vi "_Main.vi"() -> ()   [LabVIEW 2021]
uses:
  DemoApplication/DemoApplication.lvclass
  C:/Localdata/Projects/TriekselSoft/TriekselsoftApplicationFramework/Source/.Externals/Library_TAF_ApplicationFramework/MasterGUI/MasterGUI.lvclass
  .Externals/Library_TAF_ApplicationFramework/AppConfigJSON/AppConfigJSON.lvclass
  C:/Localdata/Projects/TriekselSoft/TriekselsoftApplicationFramework/Source/.Externals/Interface_TAF_IApplicationConfiguration/IApplicationConfiguration/IApplicationConfiguration.lvclass
  ErrorCreationTAF/ErrorCreationTAF.lvclass
  C:/Program Files (x86)/National Instruments/LabVIEW 2021/user.lib/_express/CustomErrorCreator/Source/ErrorCreationExecution/ErrorCreationExecution.lvclass
  .Externals/Library_TAF_TraceWindow/TraceWindow/TraceWindow.lvclass
  6e61f7a2-c992-4aa1-b06a-6e8223df94bd.vi
  cb46c3f9-39da-4d3f-bc1e-01bea614d4a3.vi
  deb2eb14-18af-4d58-82fc-a6efaabd3830.vi
  <vilib>/TriekselSoft/TracerLibrary/TracerLibrary/Tracer/protected/SendMessage.vi
  <vilib>/TriekselSoft/TracerLibrary/TracerLibrary/Tracer/protected/Timestamp.vi
  <vilib>/TriekselSoft/TracerLibrary/TracerLibrary/Tracer/Tracer_Level-Info.vi
  <vilib>/TriekselSoft/TracerLibrary/TracerLibrary/Tracer/protected/Tracer_ClassAttributes.vi
  <vilib>/TriekselSoft/TracerLibrary/TracerLibrary/Tracer/Tracer_Level-Error.vi
  .Externals/Library_TAF_ApplicationFramework/MasterGUI/MasterGUI.lvclass
  .Externals/Library_TAF_ApplicationFramework/Application/Application.lvclass
  <vilib>/TriekselSoft/TracerLibrary/TracerLibrary/Tracer/Tracer.lvclass
  <userlib>/_express/CustomErrorCreator/Source/ErrorCreationExecution/ErrorCreationExecution.lvclass
panel:
  in  "Configuration":enum16{"Default", "Mockup"}(ring)=enum."Mockup"
  out "Version":string
  out "Action":string
  out "Progress":dbl(slide) scale=0.0..1.0
  # "Application Template"
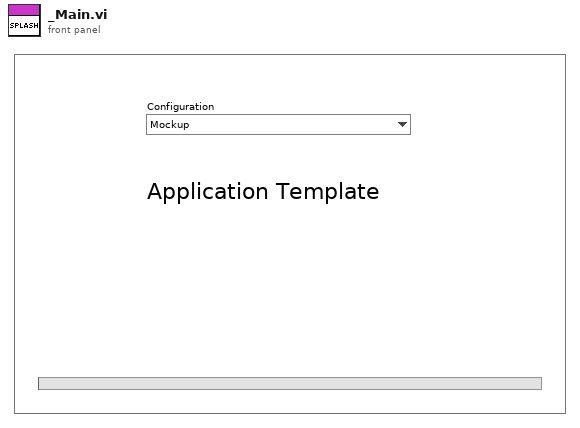
[diagram p1: front panel]
types:
  T1 = enum32{"Invalid", "Standard", "Closed", "Hidden", "Minimized", "Maximized"}
  T2 = enum32{"---START APPLICATION---", "Set Version", "Start Tracing", "Init Application", "Preload Objects", "Update Trace Items", "Create Objects", "Set External Interfaces", "Start Main GUI", "Load Presistent Data", "Show Main Window", "Hide Window", "Wait for Exit", "Save Persistent Data", "Show Window", "---EXIT APPLICATION---"}
  T3 = cluster{"DemoApplication":refnum<class "DemoApplication.lvclass">, "TraceQueue":refnum<queue>}
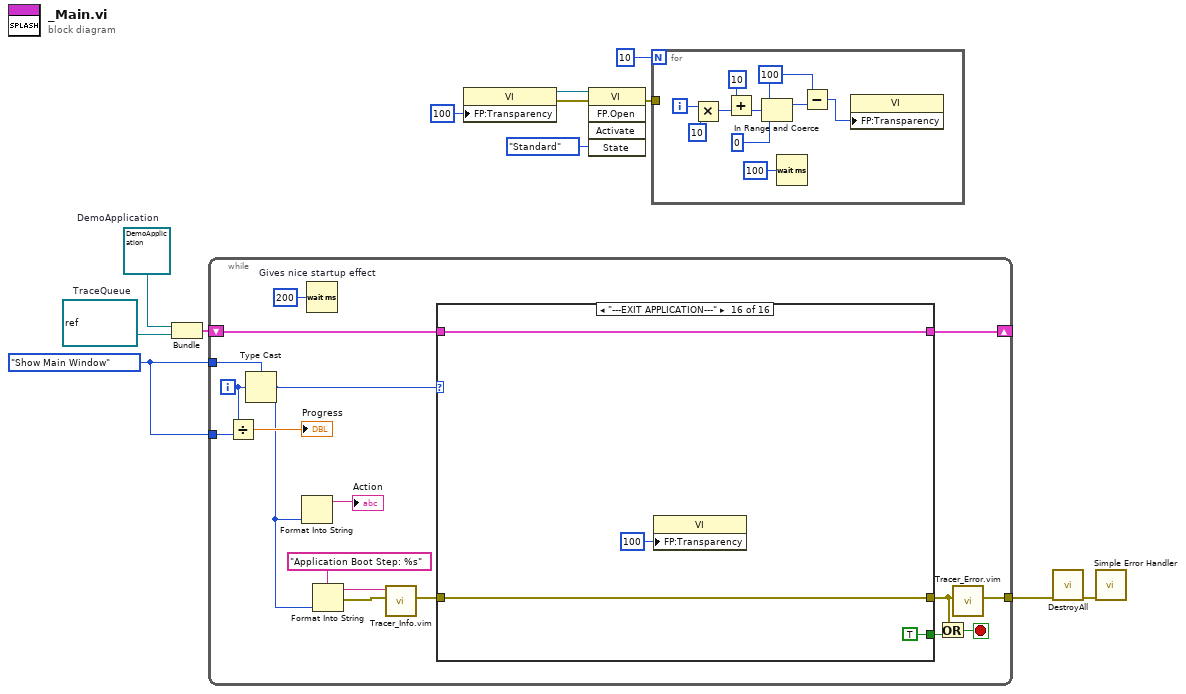
[diagram p0: block diagram]
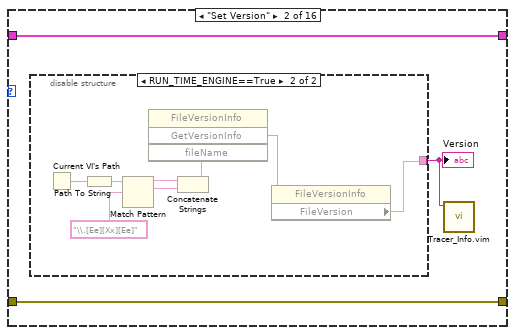
[diagram p3: hidden frame]
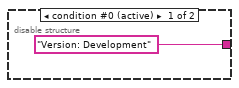
[diagram p4: hidden frame]
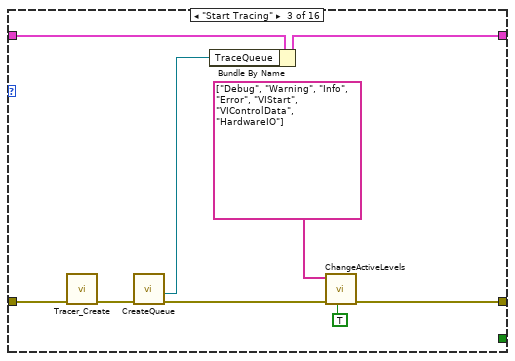
[diagram p5: hidden frame]
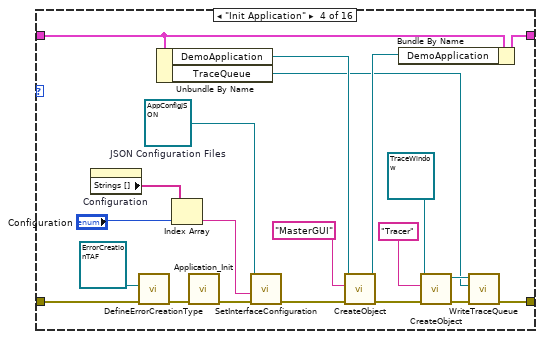
[diagram p6: hidden frame]
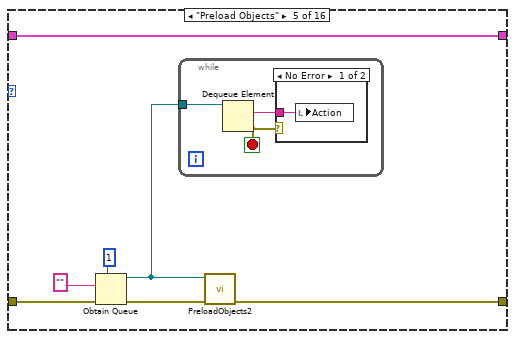
[diagram p7: hidden frame]
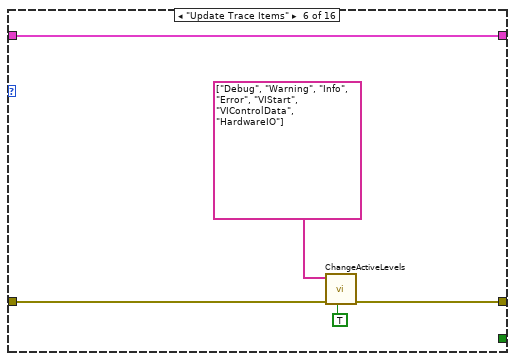
[diagram p9: hidden frame]
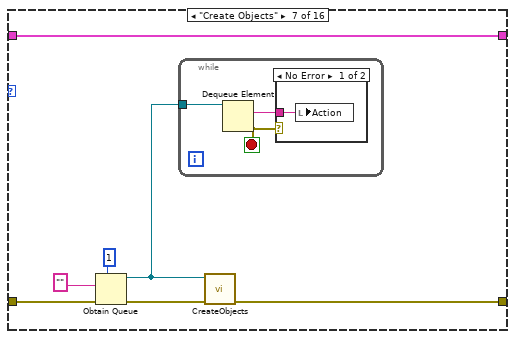
[diagram p10: hidden frame]
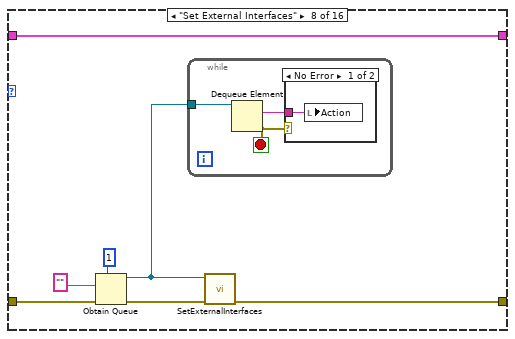
[diagram p12: hidden frame]
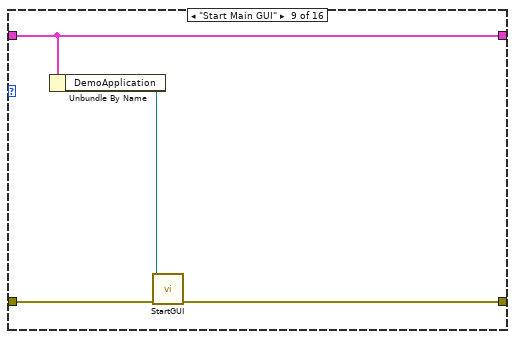
[diagram p14: hidden frame]
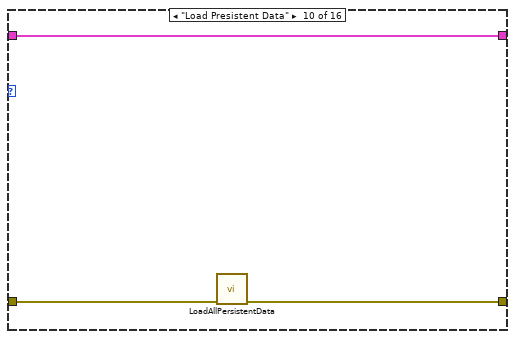
[diagram p15: hidden frame]
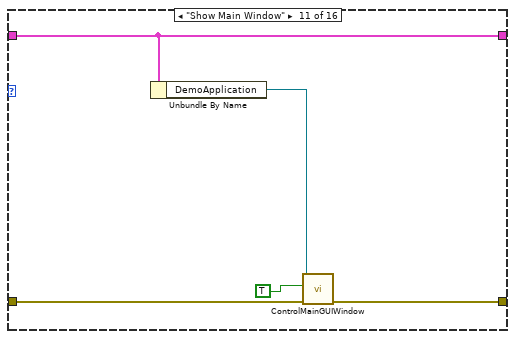
[diagram p16: hidden frame]
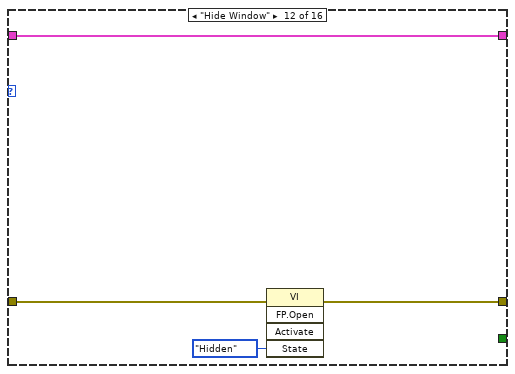
[diagram p17: hidden frame]
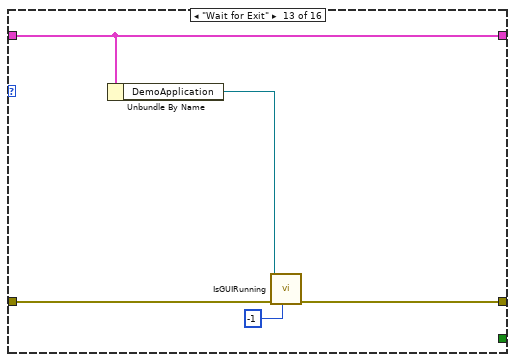
[diagram p18: hidden frame]
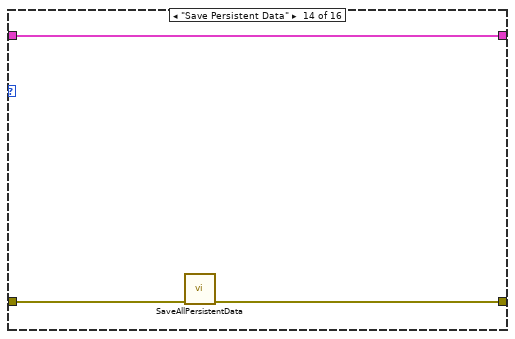
[diagram p19: hidden frame]
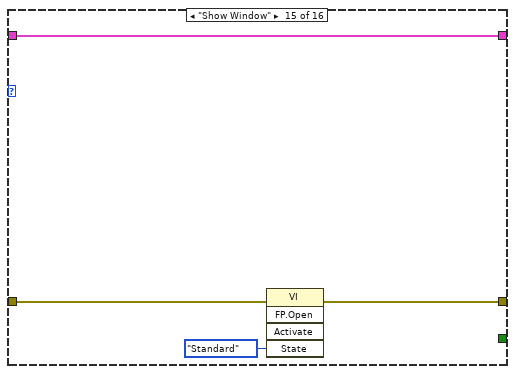
[diagram p20: hidden frame]
diagram:
  w1 = refnum<queue> refnum  # TraceQueue
  w3 = refnum<class "DemoApplication.lvclass"> refnum  # DemoApplication
  w4 = T2."Show Main Window"
  n1 = Bundle("DemoApplication"=w3, "TraceQueue"=w1) -> (w2:T3)  [unwired: 1 in]
  n2 = while {
    tunnel: w4 -> [w25]
    shift-right: [w21] -> _
    shift-left: w2 -> [w22]
    tunnel: [w28] -> w11
    tunnel: w4 -> [w15]
    i -> [w18]
    stop <- w20 stop-if-true
    n3 = Divide(x=w18, y=w15) -> (x/y=→"Progress":dbl)
    n4 = Type Cast(type=w25, x=w18) -> (*(type *) &x=w13:T2)
    n5 = Format Into String(w13) -> (resulting string=→"Action":string)  [unwired: 3 in, 1 out]
    n6 = Wait (ms) "Gives nice startup effect"(milliseconds to wait=u32 200) -> ()  [unwired: 1 out]
    n7 = Format Into String(format string="Application Boot Step: %s" ("InfoText"), w13) -> (resulting string=w23:string, error out=w27:errorcluster)  [unwired: 2 in]
    n8 = call "Tracer_Info.vim"("error in (no error)"=w27, "InfoText"=w23) -> ("error out"=w29:errorcluster)  [unwired: 9 in]
    n9 = case shown="\"---EXIT APPLICATION---\"" w13 {
      tunnel: w29 -> [w31 w34 w51 w71 w79 w88 w95 w106 w115 w118 w122 w127 w132 w135 w139 w143]
      tunnel: w22 -> [w30 w33 w46 w59 w77 w85 w93 w104 w112 w116 w120 w125 w129 w133 w137 w142]
      tunnel: [w30 w33 w45 w57 w77 w85 w93 w104 w112 w116 w120 w125 w129 w133 w137 w142] -> w21
      tunnel: [_ _ _ _ _ _ _ _ _ _ _ _ _ _ _ TRUE] -> w19
      tunnel: [w31 w34 w52 w67 w80 w89 w96 w107 w114 w117 w123 w126 w131 w134 w138 w143] -> w26
      frame "---START APPLICATION---" {
      }
      frame "Set Version" {
        n10 = disable-structure shown="RUN_TIME_ENGINE==True" {
          disable-tunnel: ["Version: Development" w36] -> w32
          frame condition #0 (active) {
          }
          frame condition #1 {
            n11 = Current VI's Path() -> (path=w39:path)
            n12 = Path To String(path=w39) -> (string=w43:string)
            n13 = Match Pattern(string=w43, regular expression="\\.[Ee][Xx][Ee]") -> (before substring=w41:string, match substring=w40:string)  [unwired: 1 in, 2 out]
            n14 = Concatenate Strings(w41, w40) -> (w42:string)
            n15 = invoke class="FileVersionInfo" method="GetVersionInfo"("fileName"=w42) -> ("GetVersionInfo"=w38:refnum<k24>)  [unwired: 3 in, 3 out]
            n16 = property class="FileVersionInfo"(reference=w38) -> ("FileVersion"=w36:string)  [unwired: 1 in, 2 out]
          }
        }
        "Version" <- w32
        n17 = call "Tracer_Info.vim"("InfoText"=w32) -> ()  [unwired: 10 in, 1 out]
      }
      frame "Start Tracing" {
        n18 = call <vilib>:"Tracer_Create.vi"("error in (no error)"=w51) -> ("error out"=w50:errorcluster)  [unwired: 10 in]
        n19 = call <vilib>:"CreateQueue.vi"("error in (no error)"=w50) -> ("error out"=w49:errorcluster, "Trace out"=w44:refnum<queue>)  [unwired: 9 in]
        n20 = Bundle By Name(cluster=w46, "TraceQueue"=w44) -> (w45:T3)
        n21 = call <vilib>:"ChangeActiveLevels.vi"("Force update"=TRUE, "error in (no error)"=w49, "ActiveLevels"=string[] ["Debug", "Warning", "Info", "Error", "VIStart", "VIControlData", "HardwareIO"] ("Active Compressed in")) -> ("error out"=w52:errorcluster)  [unwired: 8 in]
      }
      frame "Init Application" {
        w66 = refnum<class "AppConfigJSON.lvclass"> refnum  # JSON Configuration Files
        n22 = property on="Configuration" class="Enum (strict)"() -> ("Strings []"=w65:string[])  [unwired: 2 in, 2 out]
        n23 = call <userlib>:"DefineErrorCreationType.vi"("ErrorIn"=w71, "ErrorHandlingTypeClass"=refnum<class "ErrorCreationTAF.lvclass"> refnum ("ErrorCreationTAF")) -> ("ErrorOut"=w70:errorcluster)  [unwired: 9 in]
        n24 = Unbundle By Name(w59) -> ("DemoApplication"=w60:refnum<class "DemoApplication.lvclass">, "TraceQueue"=w53:refnum<queue>)
        n25 = Index Array(array=w65, index="Configuration") -> (element=w63:string)
        n26 = call "Application_Init.vi"("ErrorIn"=w70) -> ("ErrorOut"=w73:errorcluster)  [unwired: 9 in, 1 out]
        n27 = call "SetInterfaceConfiguration.vi"("ErrorIn"=w73, "StartupConfiguration"=w63, "IApplicationStructure"=w66) -> ("ErrorOut"=w72:errorcluster)  [unwired: 8 in]
        n28 = call "CreateObject.vi"("ErrorIn"=w72, "ObjectName"="MasterGUI" ("Name"), "Type"=w60) -> ("ErrorOut"=w69:errorcluster, "ObjectOut"=w58:refnum<class "DemoApplication.lvclass">)  [unwired: 7 in]
        n29 = Bundle By Name(cluster=w59, "DemoApplication"=w58) -> (w57:T3)
        n30 = call "CreateObject.vi"("ErrorIn"=w69, "ObjectName"="Tracer" ("Name"), "Type"=refnum<class "TraceWindow.lvclass"> refnum ("TraceWindow.lvlib:TraceWindow")) -> ("ErrorOut"=w68:errorcluster, "ObjectOut"=w54:refnum<class "TraceWindow.lvclass">)  [unwired: 7 in]
        n31 = call-dynamic "WriteTraceQueue.vi"("ErrorIn"=w68, "TraceQueue"=w53, "ReferenceIn"=w54) -> ("ErrorOut"=w67:errorcluster)  [unwired: 7 in, 1 out]
      }
      frame "Preload Objects" {
        n32 = Obtain Queue(max queue size (-1, unlimited)=1, element data type="", error in (no error)=w79) -> (queue out=w74:refnum<queue>, error out=w78:errorcluster)  [unwired: 2 in, 1 out]
        n33 = while {
          tunnel: w74 -> [w82]
          stop <- w83 stop-if-true
          n34 = Dequeue Element(queue=w82) -> (element=w81:string, error out=w83:errorcluster)  [unwired: 2 in, 2 out]
          n35 = case shown="No Error" w83 {
            tunnel: w81 -> [w84 _]
            frame No Error {
              n36 = local write "Action"(w84) -> ()
            }
            frame Error {
            }
          }
        }
        n37 = call "PreloadObjects2.vi"("ErrorIn"=w78, "ProgressQueue"=w74) -> ("ErrorOut"=w80:errorcluster)  [unwired: 9 in]
      }
      frame "Update Trace Items" {
        n38 = call <vilib>:"ChangeActiveLevels.vi"("Force update"=TRUE, "error in (no error)"=w88, "ActiveLevels"=string[] ["Debug", "Warning", "Info", "Error", "VIStart", "VIControlData", "HardwareIO"] ("Active Compressed in")) -> ("error out"=w89:errorcluster)  [unwired: 8 in]
      }
      frame "Create Objects" {
        n39 = Obtain Queue(max queue size (-1, unlimited)=1, element data type="", error in (no error)=w95) -> (queue out=w90:refnum<queue>, error out=w94:errorcluster)  [unwired: 2 in, 1 out]
        n40 = while {
          tunnel: w90 -> [w98]
          stop <- w99 stop-if-true
          n41 = Dequeue Element(queue=w98) -> (element=w97:string, error out=w99:errorcluster)  [unwired: 2 in, 2 out]
          n42 = case shown="No Error" w99 {
            tunnel: w97 -> [w100 _]
            frame No Error {
              n43 = local write "Action"(w100) -> ()
            }
            frame Error {
            }
          }
        }
        n44 = call "CreateObjects.vi"("ErrorIn"=w94, "ProgressQueue"=w90) -> ("ErrorOut"=w96:errorcluster)  [unwired: 9 in]
      }
      frame "Set External Interfaces" {
        n45 = Obtain Queue(max queue size (-1, unlimited)=1, element data type="", error in (no error)=w106) -> (queue out=w101:refnum<queue>, error out=w105:errorcluster)  [unwired: 2 in, 1 out]
        n46 = while {
          tunnel: w101 -> [w109]
          stop <- w110 stop-if-true
          n47 = Dequeue Element(queue=w109) -> (element=w108:string, error out=w110:errorcluster)  [unwired: 2 in, 2 out]
          n48 = case shown="No Error" w110 {
            tunnel: w108 -> [w111 _]
            frame No Error {
              n49 = local write "Action"(w111) -> ()
            }
            frame Error {
            }
          }
        }
        n50 = call "SetExternalInterfaces.vi"("ErrorIn"=w105, "ProgressQueue"=w101) -> ("ErrorOut"=w107:errorcluster)  [unwired: 9 in]
      }
      frame "Start Main GUI" {
        n51 = Unbundle By Name(w112) -> ("DemoApplication"=w113:refnum<class "DemoApplication.lvclass">)
        n52 = call-dynamic "StartGUI.vi"("ErrorIn"=w115, "ReferenceIn"=w113) -> ("ErrorOut"=w114:errorcluster)  [unwired: 8 in, 1 out]
      }
      frame "Load Presistent Data" {
        n53 = call "LoadAllPersistentData.vi"("ErrorIn"=w118) -> ("ErrorOut"=w117:errorcluster)  [unwired: 10 in]
      }
      frame "Show Main Window" {
        n54 = Unbundle By Name(w120) -> ("DemoApplication"=w119:refnum<class "DemoApplication.lvclass">)
        n55 = call "ControlMainGUIWindow.vi"("ErrorIn"=w122, "ShowProcessWindow"=TRUE, "ReferenceIn"=w119) -> ("ErrorOut"=w123:errorcluster)  [unwired: 6 in, 2 out]
      }
      frame "Hide Window" {
        n56 = invoke class="VI" method="FP.Open"(error in=w127, "State"=T1."Hidden") -> (error out=w126:errorcluster)  [unwired: 3 in, 4 out]
      }
      frame "Wait for Exit" {
        n57 = Unbundle By Name(w129) -> ("DemoApplication"=w128:refnum<class "DemoApplication.lvclass">)
        n58 = call-dynamic "IsGUIRunning.vi"("TimeoutInMs(0)"=-1 ("timeout in ms (0)"), "ErrorIn"=w132, "ReferenceIn"=w128) -> ("ErrorOut"=w131:errorcluster)  [unwired: 6 in, 2 out]
      }
      frame "Save Persistent Data" {
        n59 = call "SaveAllPersistentData.vi"("ErrorIn"=w135) -> ("ErrorOut"=w134:errorcluster)  [unwired: 10 in]
      }
      frame "Show Window" {
        n60 = invoke class="VI" method="FP.Open"(error in=w139, "State"=T1."Standard") -> (error out=w138:errorcluster)  [unwired: 3 in, 4 out]
      }
      frame "---EXIT APPLICATION---" {
        n61 = property class="VI"("FP:Transparency"=u8 100 ("Front Panel Window:Transparency")) -> ()  [unwired: 2 in, 2 out]
      }
    }
    n62 = Or(x=w26, y=w19) -> (x .or. y?=w20:bool)
    n63 = call "Tracer_Error.vim"("error in (no error)"=w26) -> ("error out"=w28:errorcluster)  [unwired: 10 in]
  }
  n64 = property class="VI"("FP:Transparency"=u8 100 ("Front Panel Window:Transparency")) -> (reference out=w8:refnum<vi>, error out=w9:errorcluster)  [unwired: 2 in]
  n65 = invoke class="VI" method="FP.Open"(reference=w8, error in=w9, "State"=T1."Standard") -> (error out=w10:errorcluster)  [unwired: 2 in, 4 out]
  n66 = for {
    N: 10 -> [_]
    tunnel: w10 -> [_]
    i -> [w147]
    w145 = 100 ("upper limit")
    n67 = Multiply(x=w147, y=10) -> (x*y=w152:i32)
    n68 = Add(x=10 ("y"), y=w152) -> (x+y=w150:i32)
    n69 = In Range and Coerce(upper limit=w145, x=w150, lower limit=0) -> (coerced(x)=w146:i32)  [unwired: 1 out]
    n70 = Wait (ms)(milliseconds to wait=u32 100) -> ()  [unwired: 1 out]
    n71 = Subtract(x=w145, y=w146) -> (x-y=w144:i32)
    n72 = property class="VI"("FP:Transparency"=w144) -> ()  [unwired: 2 in, 2 out]
  }
  n73 = call "DestroyAll.vi"("ErrorIn"=w11) -> ("ErrorOut"=w12:errorcluster)  [unwired: 10 in]
  n74 = call <vilib>:"Simple Error Handler.vi"("error in (no error)"=w12) -> ()  [unwired: 4 in, 5 out]
